vi "ActionVIOnLoad.vi"(8 "error in (no error)":errorcluster, 11 "Device Item Ref in":T1 format="%.0x") -> (0 "error out":errorcluster, 3 "Device Item Ref out":T1 format="%.0x")   [LabVIEW 2021, in "DSF System Explorer.lvlib"]
uses:
  DSF System Explorer.lvlib
  <vilib>/NI VeriStand/Custom Device API/Custom Device Item Ref.ctl
  <vilib>/NI VeriStand/Custom Device API/Custom Device API.lvlib
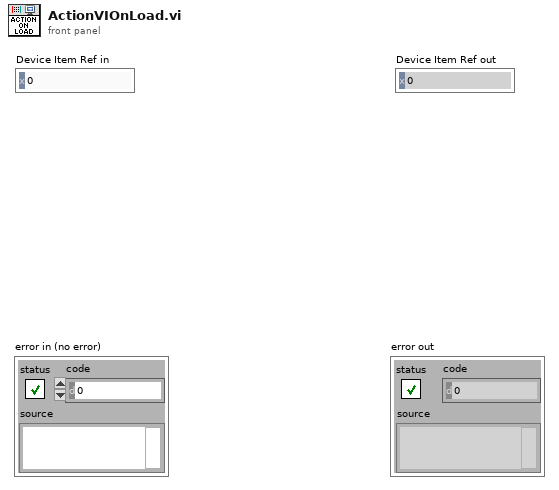
[diagram p1: front panel]
types:
  T1 = typedef "Custom Device API.lvlib/Custom Device Item Ref.ctl" = u64
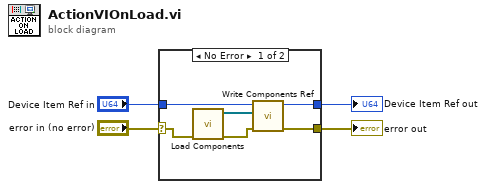
[diagram p0: block diagram]
diagram:
  n1 = case shown="No Error" "error in (no error)" {
    selector: "error in (no error)" -> [w10 w12]
    tunnel: [w7 w12] -> w3
    tunnel: "Device Item Ref in" -> [w9 w11]
    tunnel: [w8 w11] -> w1
    frame No Error {
      n2 = call "Load Components.vi"("error in (no error)"=w10) -> ("error out"=w5:errorcluster, "Components"=w6:refnum<class "Component.lvclass">[])  [unwired: 9 in]
      n3 = call "Write Components Ref.vi"("error in (no error)"=w5, "Components"=w6, "Item Ref in"=w9) -> ("error out"=w7:errorcluster, "Item Ref out"=w8:T1)  [unwired: 7 in]
    }
    frame Error {
    }
  }
  "error out" <- w3
  "Device Item Ref out" <- w1
